vi "PwmOut_read.vi"(8 "error in (no error)":errorcluster, 11 "PwmOut in":refnum<class "PwmOut.lvclass">) -> (0 "error out":errorcluster, 2 "value":dbl, 3 "PwmOut out":refnum<class "PwmOut.lvclass">)   [LabVIEW 2011, in "mbed_LVLibrary.lvlib" / "PwmOut.lvclass"]
uses:
  PwmOut.lvclass
  PwmOut.lvclass/PwmOut.ctl
  Transport Mechanisms/mbed/mbed.lvclass
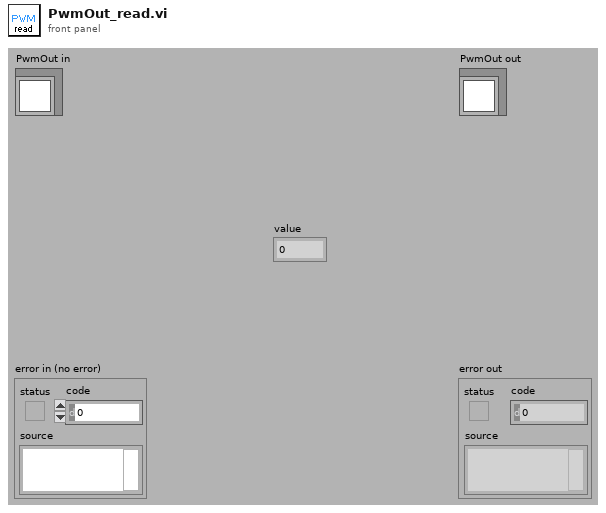
[diagram p1: front panel]
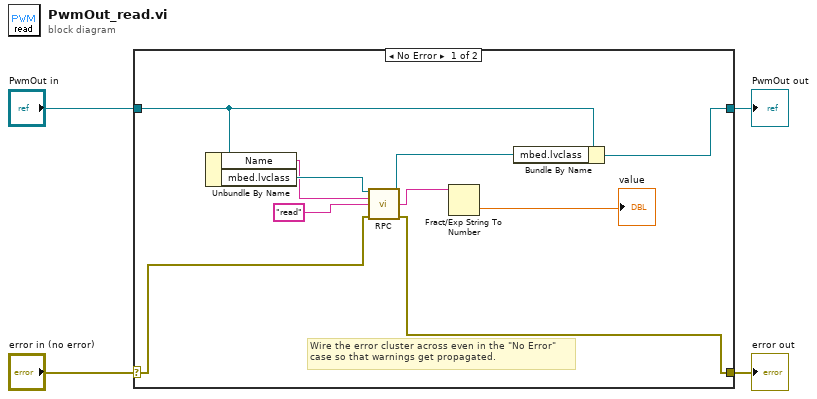
[diagram p0: block diagram]
diagram:
  n1 = case shown="No Error" "error in (no error)" {
    selector: "error in (no error)" -> [w6 w16]
    tunnel: [w5 w16] -> w3
    tunnel: [w8 w15] -> w1
    tunnel: "PwmOut in" -> [w9 w15]
    frame No Error {
      # "Wire the error cluster across even in the \"No Error\"\ncase so that warnings get propagated."
      n2 = Unbundle By Name(w9) -> ("Name"=w11:string, "mbed.lvclass"=w12:refnum<class "mbed.lvclass">)
      n3 = call-dynamic "RPC.vi"("mbed in"=w12, "Name"=w11, "method"="read", "error in (no error)"=w6) -> ("mbed out"=w7:refnum<class "mbed.lvclass">, "RPC Result"=w13:string, "error out"=w5:errorcluster)  [unwired: 9 in]
      n4 = Fract/Exp String To Number(string=w13) -> (number=→"value":dbl)  [unwired: 3 in, 1 out]
      n5 = Bundle By Name(cluster=w9, "mbed.lvclass"=w7) -> (w8:refnum<class "PwmOut.lvclass">)
    }
    frame Error {
    }
  }
  "error out" <- w3
  "PwmOut out" <- w1
